vi "Initialize Front Panel.vi"(8 "error in (no error)":errorcluster, 11 "IViewModel in":refnum<class "IViewModel.lvclass">) -> (0 "error out":errorcluster, 3 "IViewModel out":refnum<class "IViewModel.lvclass">)   [LabVIEW 2020, in "MVA Framework.lvlib" / "IViewModel.lvlib" / "IViewModel.lvclass"]
doc: "初始化前面板"
uses:
  IViewModel.lvclass
  IViewModel.lvclass/IViewModel.ctl
  IViewable/IViewable Messages/Insert Front Panel Msg/Insert Front Panel Msg.lvclass/Insert Front Panel Msg.ctl
  <vilib>/ActorFramework/Message Enqueuer/Message Enqueuer.lvclass/Message Enqueuer.ctl
  <vilib>/ActorFramework/Message Enqueuer/Enqueue.vi
  IViewable/IViewable Messages/Insert Front Panel Msg/Insert Front Panel Msg.lvclass
  C:/Program Files/National Instruments/LabVIEW 2020/vi.lib/ActorFramework/Message/Message.lvclass
  <vilib>/ActorFramework/Message Priority Queue/Priority Enqueue.vi
  IViewManager/IViewManager/IViewManager.lvclass
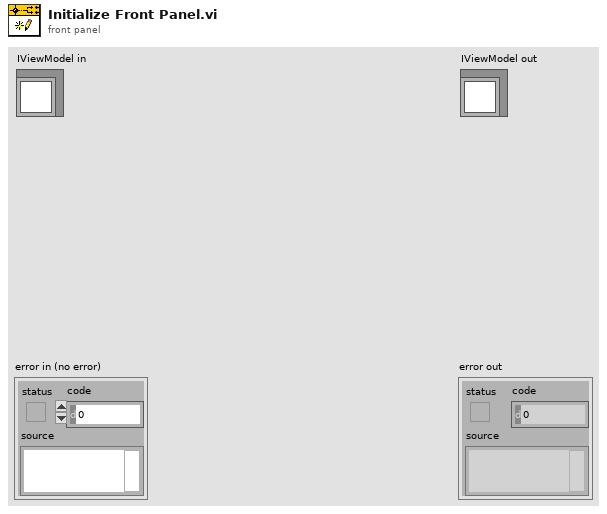
[diagram p1: front panel]
types:
  T1 = typedef "MVA Framework.lvlib/IViewable.lvlib/ProtectedSubpanel.lvclass/Protected Subpanel Reference.ctl" = refnum<data-value>
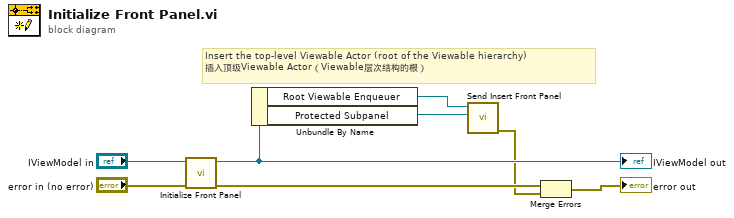
[diagram p0: block diagram]
diagram:
  # "Insert the top-level Viewable Actor (root of the Viewable hierarchy)\n插入顶级Viewable Actor（Viewable层次结构的根）"
  n1 = call-parent "Initialize Front Panel.vi"("error in (no error)"="error in (no error)", "IViewable in"="IViewModel in") -> ("error out"=w8:errorcluster, "IViewable out"=w4:refnum<class "IViewModel.lvclass">)  [unwired: 8 in]
  "IViewModel out" <- w4
  n2 = Unbundle By Name(w4) -> ("Root Viewable Enqueuer"=w3:refnum<class "Message Enqueuer.lvclass">, "Protected Subpanel"=w5:T1)
  n3 = call "Send Insert Front Panel.vi"("Protected Subpanel"=w5, "Message Enqueuer"=w3) -> ("error out"=w1:errorcluster)  [unwired: 8 in, 1 out]
  n4 = Merge Errors(w8, w1) -> (→"error out":errorcluster)
